vi "KlingerV2 Init.vi"(0 "VISA_Res":refnum<visa-resource-name>="GPIB0::12::INSTR", 3 "error in":errorcluster, 4 "Axe":u8(ring) items=["W", "X", "Y", "Z"]) -> (5 "Message D'erreur":string, 6 "Ind Comm":string caption="Indicateur de commande", 7 "error out":errorcluster)   [LabVIEW 2012]
doc: "Ce VI Initialise les différentes options du contrôlleur. Les options vitesses et accélération sont appliquées sur l'axe courant seulement."
uses:
  <userlib>/KlingerV2/KlingerV2 Params.ctl
panel:
  in  "StatusOpt":T1={"AXIS MOVING"=TRUE, "W & X TRAVEL LIMIT"=TRUE, "Y & Z TRAVEL LIMIT"=TRUE, "INPUT BITS VALUE"=TRUE, "W  POSITION"=TRUE, "X  POSITION"=TRUE, "Y  POSITION"=TRUE, "Z  POSITION"=TRUE} caption="Status Report Options"
  out "Statut":bool
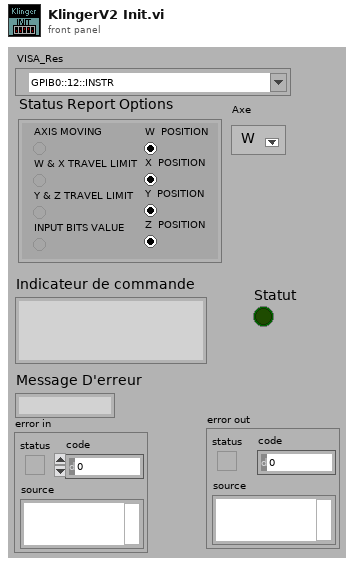
[diagram p1: front panel]
types:
  T1 = cluster{"AXIS MOVING":bool, "W & X TRAVEL LIMIT":bool, "Y & Z TRAVEL LIMIT":bool, "INPUT BITS VALUE":bool, "W  POSITION":bool, "X  POSITION":bool, "Y  POSITION":bool, "Z  POSITION":bool}
  T2 = typedef "KlingerV2 Params.ctl" = enum16{"Type", "Origine", "Encodeur", "TypeMouv", "FactConv", "Nom", "CorrParams", "KlingCtrlPar", "Speed", "Acc", "Avance", "Tous"}
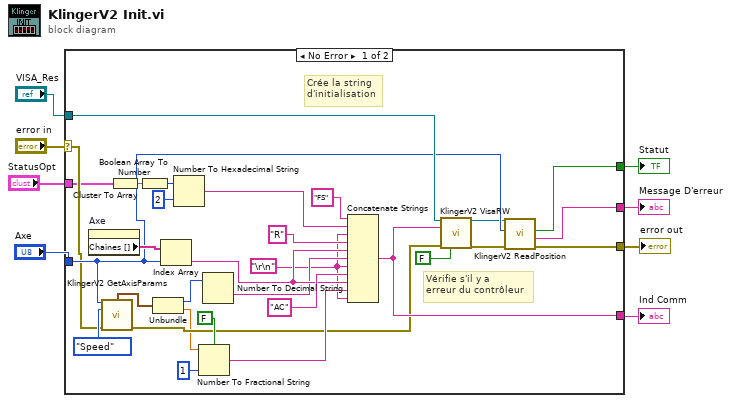
[diagram p0: block diagram]
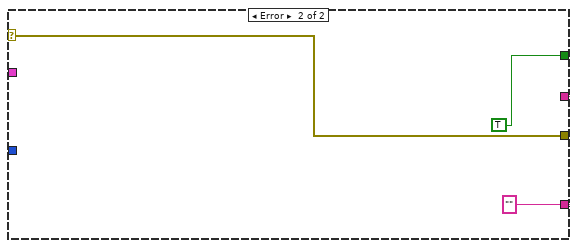
[diagram p2: hidden frame]
diagram:
  n1 = case shown="No Error" "error in" {
    selector: "error in" -> [w23 w41]
    tunnel: [w28 w39] -> w8
    tunnel: [w31 TRUE ("Statut")] -> w5
    tunnel: [w32 w41] -> w7
    tunnel: "Axe" -> [w25 _]
    tunnel: [w30 w39] -> w3
    tunnel: "VISA_Res" -> [w26 _]
    tunnel: "StatusOpt" -> [w14 _]
    frame No Error {
      w9 = "\r\n"
      # "Vérifie s'il y a \nerreur du contrôleur"
      # "Crée la string\nd'initialisation"
      n2 = property on="Axe" class="Ring (strict)"() -> ("Chaînes []"=w34:string[])  [unwired: 2 in, 2 out]
      n3 = call <userlib>:"KlingerV2 GetAxisParams.vi"("Axe"=w25, "Param"=KlingerV2_Params."Speed", "error in"=w23) -> ("Speed"=w21:cluster{"Vitesse":i32, "Accel":dbl}, "error out"=w22:errorcluster)  [unwired: 3 in, 8 out]
      n4 = Cluster To Array(cluster=w14) -> (array=w15:bool[])
      n5 = Boolean Array To Number(Boolean array=w15) -> (number=w16:u32)
      n6 = Unbundle(w21) -> ("Vitesse"=w20:i32, "Accel"=w19:dbl)
      n7 = Index Array(array=w34, index=w25) -> (element=w33:string)
      n8 = Number To Hexadecimal String(1:i16 2 ("width (-)"), 2:w16) -> (0:w13:string)
      n9 = Number To Fractional String(use system decimal point (T)=FALSE, number=w19, precision (6)=i16 1) -> (F-format string=w36:string)  [unwired: 1 in]
      n10 = Number To Decimal String(number=w20) -> (decimal integer string=w10:string)  [unwired: 1 in]
      n11 = Concatenate Strings("FS", w13, w9, "R", w33, w10, w9, "AC", w33, w36, w9) -> (w28:string)
      n12 = call <userlib>:"KlingerV2 VisaRW.vi"("VISA Rsrc"=w26, "ChaineCom"=w28, "error in (no error)"=w22, "Lecture?(T)"=FALSE) -> ("VISA Rsrc Out"=w18:refnum<visa-resource-name>, "error out"=w29:errorcluster)  [unwired: 7 in, 3 out]
      n13 = call <userlib>:"KlingerV2 ReadPosition.vi"("error in"=w29, "Axe"=w25, "VISA Rsrc"=w18) -> ("error out"=w32:errorcluster, "Cont Error"=w30:string, "Statut"=w31:bool)  [unwired: 2 in, 4 out]
    }
    frame Error {
      w39 = ""
    }
  }
  "error out" <- w7
  "Ind Comm" <- w8
  "Statut" <- w5
  "Message D'erreur" <- w3
